vi "UnregisterImagePtr.vi"(8 "error in":errorcluster, 10 "ImagePointer":T1 {"ImagePointer" format="%.0x"}, 11 "Image Reference In":T3) -> (0 "error out":errorcluster, 3 "Image Reference Out":T3)   [LabVIEW 2020, in "OpenLvVision_Image.lvlib" / "DataAccess.lvlib"]
doc: "Provides the image's memory pointer and alignment details."
uses:
  Management/TypeDef/Image.ctl
  DataAccess.lvlib
  TypeDef/PixelPointer.ctl
  Management/Management.lvlib
  Management/TypeDef/ImageType.ctl
  TypeDef/ImagePointer.ctl
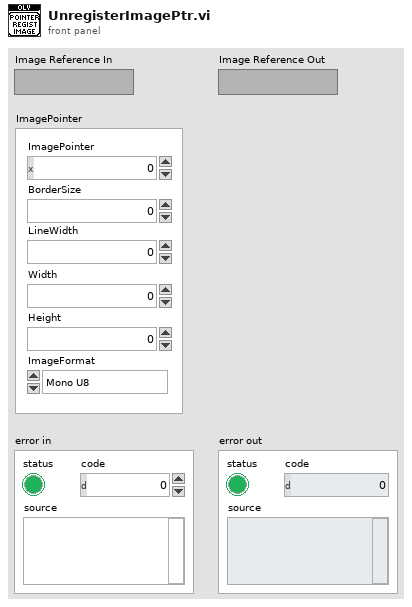
[diagram p1: front panel]
types:
  T1 = typedef "OpenLvVision_Image.lvlib/DataAccess.lvlib/ImagePointer.ctl" = cluster{"ImagePointer":u64, "BorderSize":i32, "LineWidth":i32, "Width":i32, "Height":i32, "ImageFormat":T2}
  T2 = typedef "OpenLvVision_Image.lvlib/Management.lvlib/ImageType.ctl" = enum16{"Mono U8", "Mono U16", "Mono I16", "Mono SGL", "Color U32", "Color U64"}
  T3 = typedef "OpenLvVision_Image.lvlib/Management.lvlib/Image.ctl" = refnum<image>
  T4 = typedef "OpenLvVision_Image.lvlib/DataAccess.lvlib/PixelPointer.ctl" = cluster{"Image Border Size":i32, "Pixel Pointer":u64, "LineWidth":i32, "PixelSize_Bytes":i32, "TransferMaxSize":i32}
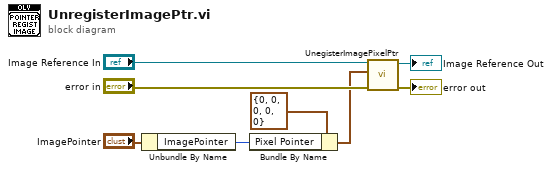
[diagram p0: block diagram]
diagram:
  n1 = Unbundle By Name("ImagePointer") -> ("ImagePointer"=w1:u64)
  n2 = Bundle By Name(cluster=T4 {"Image Border Size"=0, "Pixel Pointer"=0, "LineWidth"=0, "PixelSize_Bytes"=0, "TransferMaxSize"=0} ("PixelPointer"), "Pixel Pointer"=w1) -> (w3:T4)
  n3 = call "UnegisterImagePixelPtr.vi"("error in"="error in", "PixelPointer"=w3, "Image Reference In"="Image Reference In") -> ("error out"=→"error out":errorcluster, "Image Reference Out"=→"Image Reference Out":T3)  [unwired: 7 in]
